vi "Initialization_T_B_ver1.1.vi"(1 "output cluster":T1={"Main Sweep"=0, "Steps Config:"={"total points:"=0, "Step Delay (s)"=0.0, "Ini Delay (s)"=0.0, "# of steps:"=0}, "Temperature Control (ITC 503):"={"GPIB ADR"=0, "Change Heater?"={"Heater?"=FALSE, "Heater"=0}, "Change Temp?"={"Change T?"=FALSE, "Set T (K)"=0.0}, "Cluster"={"Heat Auto?"=FALSE, "Manual Heat?"=FALSE, "Heater (%)"=0.0}, "Change PID?"={"Change PID?"=FALSE, "P"=0.0, "I"=0.0, "D"=0.0}, "Change Para?"=FALSE, "Sensor"=1}, "Temperature Control (LS 340):"={"GPIB ADR"=0, "From (K)"=0.0, "To (K)"=0.0, "Rate (K/min)"=0.0, "Delta T (0.08K)"=0.0, "Temp. Header"="", "T Display Control"={"Ch B"=FALSE, "Ch C"=FALSE, "Ch D"=FALSE}}, "Magnet Control (IPS 120-10)"={"Action"=0, "Standby (s)"=0.0, "Heater on (s)"=0.0, "Sweep Setup "=[], "GPIB ADR"=0, "Change Para?"=FALSE}, "Keithley 6221 :"=[], "Measuring Instruments : "=[], "Lock-In SR7265 :"=[], "Deascription of \nthis measurement"="", "Instruments Config:"=[], "LS372 Bridge : 2"=[{"GPIB"=0, "Excitation"=0, "Autorange?"=FALSE, "Range"=0, "Current"=0, "Voltage"=0, "DataHeader"="Rx;Ry"}], "Magnet Control (CS4) 2"={"Action"=1, "Standby (s)"=0.0, "Heater on (s)"=300.0, "Sweep Setup "=[], "GPIB ADR"=0, "Change Para?"=FALSE}} {"Magnet Control (CS4) 2"."GPIB ADR" items=["None"=0, "10"=10]; "Magnet Control (CS4) 2"."Sweep Setup"."Rate in Range (T/min)" min=0.001 max=0.5 step=0.001; "Magnet Control (CS4) 2"."Sweep Setup"."Hold(min)" min=0.0; "Magnet Control (CS4) 2"."Sweep Setup"."Set Point (T)" min=-9.0 max=9.0 step=0.001; "Magnet Control (CS4) 2"."Action" items=["Up", "Down", "Pause", "Zero"]; "LS372 Bridge : 2"."Voltage" items=["2.00 uV"=1, "6.32 uV"=2, "20.0 uV"=3, "63.2 uV"=4, "200 uV"=5, "632 uV"=6, "2.0 mV"=7, "6.32 mV"=8]; "LS372 Bridge : 2"."Current" items=["1.00 pA"=1, "3.16 pA"=2, "10.0 pA"=3, "31.6 pA"=4, "100 pA"=5, "316 pA"=6, "1.00 nA"=7, "3.16 nA"=8, "10 nA"=9, "31.6 nA"=10, "100 nA"=11, "316 nA"=12, "1.00 uA"=13, "3.16 uA"=14, "10.0 uA"=15, "31.6 uA"=16, "100 uA"=17, "316 uA"=18, "1.00 mA"=19, "3.16 mA"=20, "10.0 mA"=21, "31.6 mA"=22]; "LS372 Bridge : 2"."Range" items=["2.0 m"=1, "6.32 m"=2, "20.0 m"=3, "63.2 m"=4, "200 m"=5, "632 m"=6, "2.00"=7, "6.32"=8, "20.0"=9, "63.2"=10, "200"=11, "632"=12, "2.00 k"=13, "6.32 k"=14, "20.0 k"=15, "63.2 k"=16, "200 k"=17, "632 k"=18, "2.00 M"=19, "6.32 M"=20, "20.0 M"=21, "63.2 M"=22]; "LS372 Bridge : 2"."Excitation" items=["Voltage", "Current"]; "LS372 Bridge : 2"."GPIB" items=["None"=0, "9"=9]; "Main Sweep" items=["Time", "DC Current", "Delta Current", "Pulse Delta Current", "Sine Current", "Lock-in Vosc"]; "Temperature Control (ITC 503):"."Sensor" items=["T2", "T3"]; "Magnet Control (IPS 120-10)"."Action" items=["Hold", "To Set point", "To Zero", "Clamp"]; "Keithley 6221 :"."Sweep Mode" items=["Linear", "Log", "Exp", "Inverse", "Manual"]}, 5 "Measure with H/T sweep?":bool, 6 "error in (no error)":errorcluster, 7 "First run?":bool, 8 "Last run?":bool, 9 "B Field Display Tex Array":refnum<vi>[](array[refnum]), 10 "Temp. Display Ref Array":refnum<vi>[](array[refnum])) -> (0 "error out":errorcluster, 2 "output cluster 2":T1={"Main Sweep"=0, "Steps Config:"={"total points:"=0, "Step Delay (s)"=0.0, "Ini Delay (s)"=0.0, "# of steps:"=0}, "Temperature Control (ITC 503):"={"GPIB ADR"=0, "Change Heater?"={"Heater?"=FALSE, "Heater"=0}, "Change Temp?"={"Change T?"=FALSE, "Set T (K)"=0.0}, "Cluster"={"Heat Auto?"=FALSE, "Manual Heat?"=FALSE, "Heater (%)"=0.0}, "Change PID?"={"Change PID?"=FALSE, "P"=0.0, "I"=0.0, "D"=0.0}, "Change Para?"=FALSE, "Sensor"=1}, "Temperature Control (LS 340):"={"GPIB ADR"=0, "From (K)"=0.0, "To (K)"=0.0, "Rate (K/min)"=0.0, "Delta T (0.08K)"=0.0, "Temp. Header"="", "T Display Control"={"Ch B"=FALSE, "Ch C"=FALSE, "Ch D"=FALSE}}, "Magnet Control (IPS 120-10)"={"Action"=0, "Standby (s)"=0.0, "Heater on (s)"=0.0, "Sweep Setup "=[], "GPIB ADR"=0, "Change Para?"=FALSE}, "Keithley 6221 :"=[], "Measuring Instruments : "=[], "Lock-In SR7265 :"=[], "Deascription of \nthis measurement"="", "Instruments Config:"=[], "LS372 Bridge : 2"=[{"GPIB"=0, "Excitation"=0, "Autorange?"=FALSE, "Range"=0, "Current"=0, "Voltage"=0, "DataHeader"="Rx;Ry"}], "Magnet Control (CS4) 2"={"Action"=1, "Standby (s)"=0.0, "Heater on (s)"=300.0, "Sweep Setup "=[], "GPIB ADR"=0, "Change Para?"=FALSE}} {"Magnet Control (CS4) 2"."GPIB ADR" items=["None"=0, "25"=25]; "Magnet Control (CS4) 2"."Sweep Setup"."Rate in Range (T/min)" min=0.001 max=0.5 step=0.001; "Magnet Control (CS4) 2"."Sweep Setup"."Hold(min)" min=0.0; "Magnet Control (CS4) 2"."Sweep Setup"."Set Point (T)" min=-9.0 max=9.0 step=0.001; "Magnet Control (CS4) 2"."Action" items=["Up", "Down", "Pause", "Zero"]; "LS372 Bridge : 2"."Voltage" items=["2.00 uV"=1, "6.32 uV"=2, "20.0 uV"=3, "63.2 uV"=4, "200 uV"=5, "632 uV"=6, "2.0 mV"=7, "6.32 mV"=8]; "LS372 Bridge : 2"."Current" items=["1.00 pA"=1, "3.16 pA"=2, "10.0 pA"=3, "31.6 pA"=4, "100 pA"=5, "316 pA"=6, "1.00 nA"=7, "3.16 nA"=8, "10 nA"=9, "31.6 nA"=10, "100 nA"=11, "316 nA"=12, "1.00 uA"=13, "3.16 uA"=14, "10.0 uA"=15, "31.6 uA"=16, "100 uA"=17, "316 uA"=18, "1.00 mA"=19, "3.16 mA"=20, "10.0 mA"=21, "31.6 mA"=22]; "LS372 Bridge : 2"."Range" items=["2.0 m"=1, "6.32 m"=2, "20.0 m"=3, "63.2 m"=4, "200 m"=5, "632 m"=6, "2.00"=7, "6.32"=8, "20.0"=9, "63.2"=10, "200"=11, "632"=12, "2.00 k"=13, "6.32 k"=14, "20.0 k"=15, "63.2 k"=16, "200 k"=17, "632 k"=18, "2.00 M"=19, "6.32 M"=20, "20.0 M"=21, "63.2 M"=22]; "LS372 Bridge : 2"."Excitation" items=["Voltage", "Current"]; "LS372 Bridge : 2"."GPIB" items=["None"=0, "9"=9]; "Main Sweep" items=["Time", "DC Current", "Delta Current", "Pulse Delta Current", "Sine Current", "Lock-in Vosc"]; "Temperature Control (ITC 503):"."Sensor" items=["T2", "T3"]; "Magnet Control (IPS 120-10)"."Action" items=["Hold", "To Set point", "To Zero", "Clamp"]; "Keithley 6221 :"."Sweep Mode" items=["Linear", "Log", "Exp", "Inverse", "Manual"]}, 3 "Title Array":string[](array[string]), 4 "Comments String":string)   [LabVIEW 2012]
doc: "Initialize the temperature (LS336)"
panel:
  out "BField Display Cluster":cluster{"B":dbl} {"B" min=0.0 format="%_5f"}
  out "B Set Pt (T)":dbl format="%_5g"
  out "B Rate (T/min)":dbl format="%_5g"
  out "Temp Graph 2":dbl[][](graph)=[[348.0650696299951, 348.0650696299951, 348.0650696299951, 348.0650696299951, 348.0650696299951, 348.0650696299951, 348.0650696299951, 348.0650696299951, 348.0650696299951, 348.0650696299951, 348.0650696299951, 348.0650696299951, 348.0650696299951, 348.0650696299951, 348.0650696299951], [349.0, 349.0, 349.0, 349.0, 349.0, 349.0, 349.0, 349.0, 349.0, 349.0, 349.0, 349.0, 349.0, 349.0, 349.0], [347.994, 347.998, 348.007, 348.013, 348.031, 348.047, 348.071, 348.073, 348.076, 348.088, 348.106, 348.11, 348.113, 348.121, 348.128], [349.08, 349.08, 349.08, 349.08, 349.08, 349.08, 349.08, 349.08, 349.08, 349.08, 349.08, 349.08, 349.08, 349.08, 349.08], [348.92, 348.92, 348.92, 348.92, 348.92, 348.92, 348.92, 348.92, 348.92, 348.92, 348.92, 348.92, 348.92, 348.92, 348.92]]
  out "StartTime":u32
  in  "Skip":bool
  out "Time 2":string
  in  "Timeout (min)":u32=30
  out "Reach to set pt?":bool
  out "T Rate (K/min)":dbl format="%_5g"
  out "T Set Pt (K)":dbl format="%_5g"
  out "Temp Display Cluster":cluster{"RMS T:":dbl, "T STD":dbl, "T":dbl} {"T STD" min=0.0 format="%8.4f"; "T" min=0.0 format="%_5f"; "RMS T:" format="%_5g"}
  out "Temp Graph":dbl[][](graph)=[[348.0650696299951, 348.0650696299951, 348.0650696299951, 348.0650696299951, 348.0650696299951, 348.0650696299951, 348.0650696299951, 348.0650696299951, 348.0650696299951, 348.0650696299951, 348.0650696299951, 348.0650696299951, 348.0650696299951, 348.0650696299951, 348.0650696299951], [349.0, 349.0, 349.0, 349.0, 349.0, 349.0, 349.0, 349.0, 349.0, 349.0, 349.0, 349.0, 349.0, 349.0, 349.0], [347.994, 347.998, 348.007, 348.013, 348.031, 348.047, 348.071, 348.073, 348.076, 348.088, 348.106, 348.11, 348.113, 348.121, 348.128], [349.08, 349.08, 349.08, 349.08, 349.08, 349.08, 349.08, 349.08, 349.08, 349.08, 349.08, 349.08, 349.08, 349.08, 349.08], [348.92, 348.92, 348.92, 348.92, 348.92, 348.92, 348.92, 348.92, 348.92, 348.92, 348.92, 348.92, 348.92, 348.92, 348.92]]
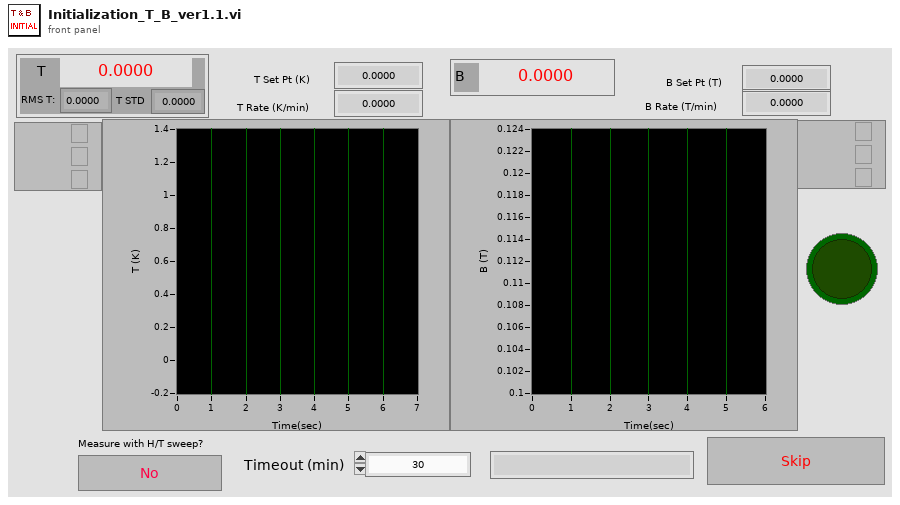
[diagram p1: front panel]
types:
  T1 = cluster{"Main Sweep":u8, "Steps Config:":cluster{"total points:":u32, "Step Delay (s)":dbl, "Ini Delay (s)":dbl, "# of steps:":u32}, "Temperature Control (ITC 503):":cluster{"GPIB ADR":u16, "Change Heater?":cluster{"Heater?":bool, "Heater":u8}, "Change Temp?":cluster{"Change T?":bool, "Set T (K)":dbl}, "Cluster":cluster{"Heat Auto?":bool, "Manual Heat?":bool, "Heater (%)":dbl}, "Change PID?":cluster{"Change PID?":bool, "P":dbl, "I":dbl, "D":dbl}, "Change Para?":bool, "Sensor":u16}, "Temperature Control (LS 340):":cluster{"GPIB ADR":u16, "From (K)":dbl, "To (K)":dbl, "Rate (K/min)":dbl, "Delta T (0.08K)":dbl, "Temp. Header":string, "T Display Control":cluster{"Ch B":bool, "Ch C":bool, "Ch D":bool}}, "Magnet Control (IPS 120-10)":cluster{"Action":u16, "Standby (s)":dbl, "Heater on (s)":dbl, "Sweep Setup ":cluster{"Set Point (T)":dbl, "Set Rate(T/min)":dbl, "Hold(min)":dbl}[], "GPIB ADR":u16, "Change Para?":bool}, "Keithley 6221 :":cluster{"Delta mode":bool, "Const I":bool, "Pulse Delta mode":bool, "Sine Wave Mode":bool, "From I_HI (A)":dbl, "From I (A)":dbl, "I_LO (A)":dbl, "From I_H (A)":dbl, "I_L (A)":dbl, "Freq (Hz)":dbl, "From I_Sin (A)":dbl, "DC Offset (A)":dbl, "Delay Time (s)":dbl, "Pulse Width (s)":dbl, "Delay (s)":dbl, "To I (A)":dbl, "ASymmetric?":bool, "To I_HI (A)":dbl, "To I_H (A)":dbl, "To I_Sin (A)":dbl, "GPIB ADR":u16, "Sweep Mode":u8, "Delta Unit":string, "2182A range (V)":dbl, "6221 Compliance (V)":dbl}[], "Measuring Instruments : ":cluster{"GPIB Bus":dbl, "GPIB Addr":dbl, "Instrument":enum16{"None", "HP34401DMM", "Lockin 7265", "HP3456/7A", "HP3478A", "HP3325FG", "Keithley2182A"}, "Instru Header":string}[], "Lock-In SR7265 :":cluster{"GPIB ADR":u16, "From":dbl, "To":dbl, "Header(;)":string, "Sweep Mode":u8}[], "Deascription of \nthis measurement":string, "Instruments Config:":string[][], "LS372 Bridge : 2":cluster{"GPIB":u16, "Excitation":u16, "Autorange?":bool, "Range":u16, "Current":u16, "Voltage":u16, "DataHeader":string}[], "Magnet Control (CS4) 2":cluster{"Action":u16, "Standby (s)":dbl, "Heater on (s)":dbl, "Sweep Setup ":cluster{"Set Point (T)":dbl, "Hold(min)":dbl, "Rate in Range (T/min)":dbl[]}[], "GPIB ADR":u16, "Change Para?":bool}}
  T2 = cluster{"GPIB ADR":u16, "Change Heater?":cluster{"Heater?":bool, "Heater":u8}, "Change Temp?":cluster{"Change T?":bool, "Set T (K)":dbl}, "Cluster":cluster{"Heat Auto?":bool, "Manual Heat?":bool, "Heater (%)":dbl}, "Change PID?":cluster{"Change PID?":bool, "P":dbl, "I":dbl, "D":dbl}, "Change Para?":bool, "Sensor":u16}
  T3 = cluster{"Action":u16, "Standby (s)":dbl, "Heater on (s)":dbl, "Sweep Setup ":cluster{"Set Point (T)":dbl, "Set Rate(T/min)":dbl, "Hold(min)":dbl}[], "GPIB ADR":u16, "Change Para?":bool}
  T4 = cluster{"GPIB ADR":u16, "From (K)":dbl, "To (K)":dbl, "Rate (K/min)":dbl, "Delta T (0.08K)":dbl, "Temp. Header":string, "T Display Control":cluster{"Ch B":bool, "Ch C":bool, "Ch D":bool}}
  T5 = cluster{"Action":u16, "Standby (s)":dbl, "Heater on (s)":dbl, "Sweep Setup ":cluster{"Set Point (T)":dbl, "Hold(min)":dbl, "Rate in Range (T/min)":dbl[]}[], "GPIB ADR":u16, "Change Para?":bool}
  T6 = cluster{"RMS":dbl, "STD":dbl, "Current value":dbl}
  T7 = cluster{"Com Port":i32, "ISOBUS Address":i32, "GPIB Address":i16, "Communication":enum16{"RS232", "ISOBUS", "GPIB", "Gateway"}}
  T8 = cluster{"GPIB ADR":u16, "Change Heater?":cluster{"Change Heater?":bool, "Heater":u8}, "Change Temp?":cluster{"Change Temp?":bool, "Set Temp (K)":dbl}, "Cluster":cluster{"Heat Auto?":bool, "Manual Heat?":bool, "Heater Manual (%)":dbl}, "Change PID?":cluster{"Change PID?":bool, "Proportional":dbl, "Integral":dbl, "Derivative":dbl}, "Change Para?":bool, "ITC503 Control Sensor":u16}
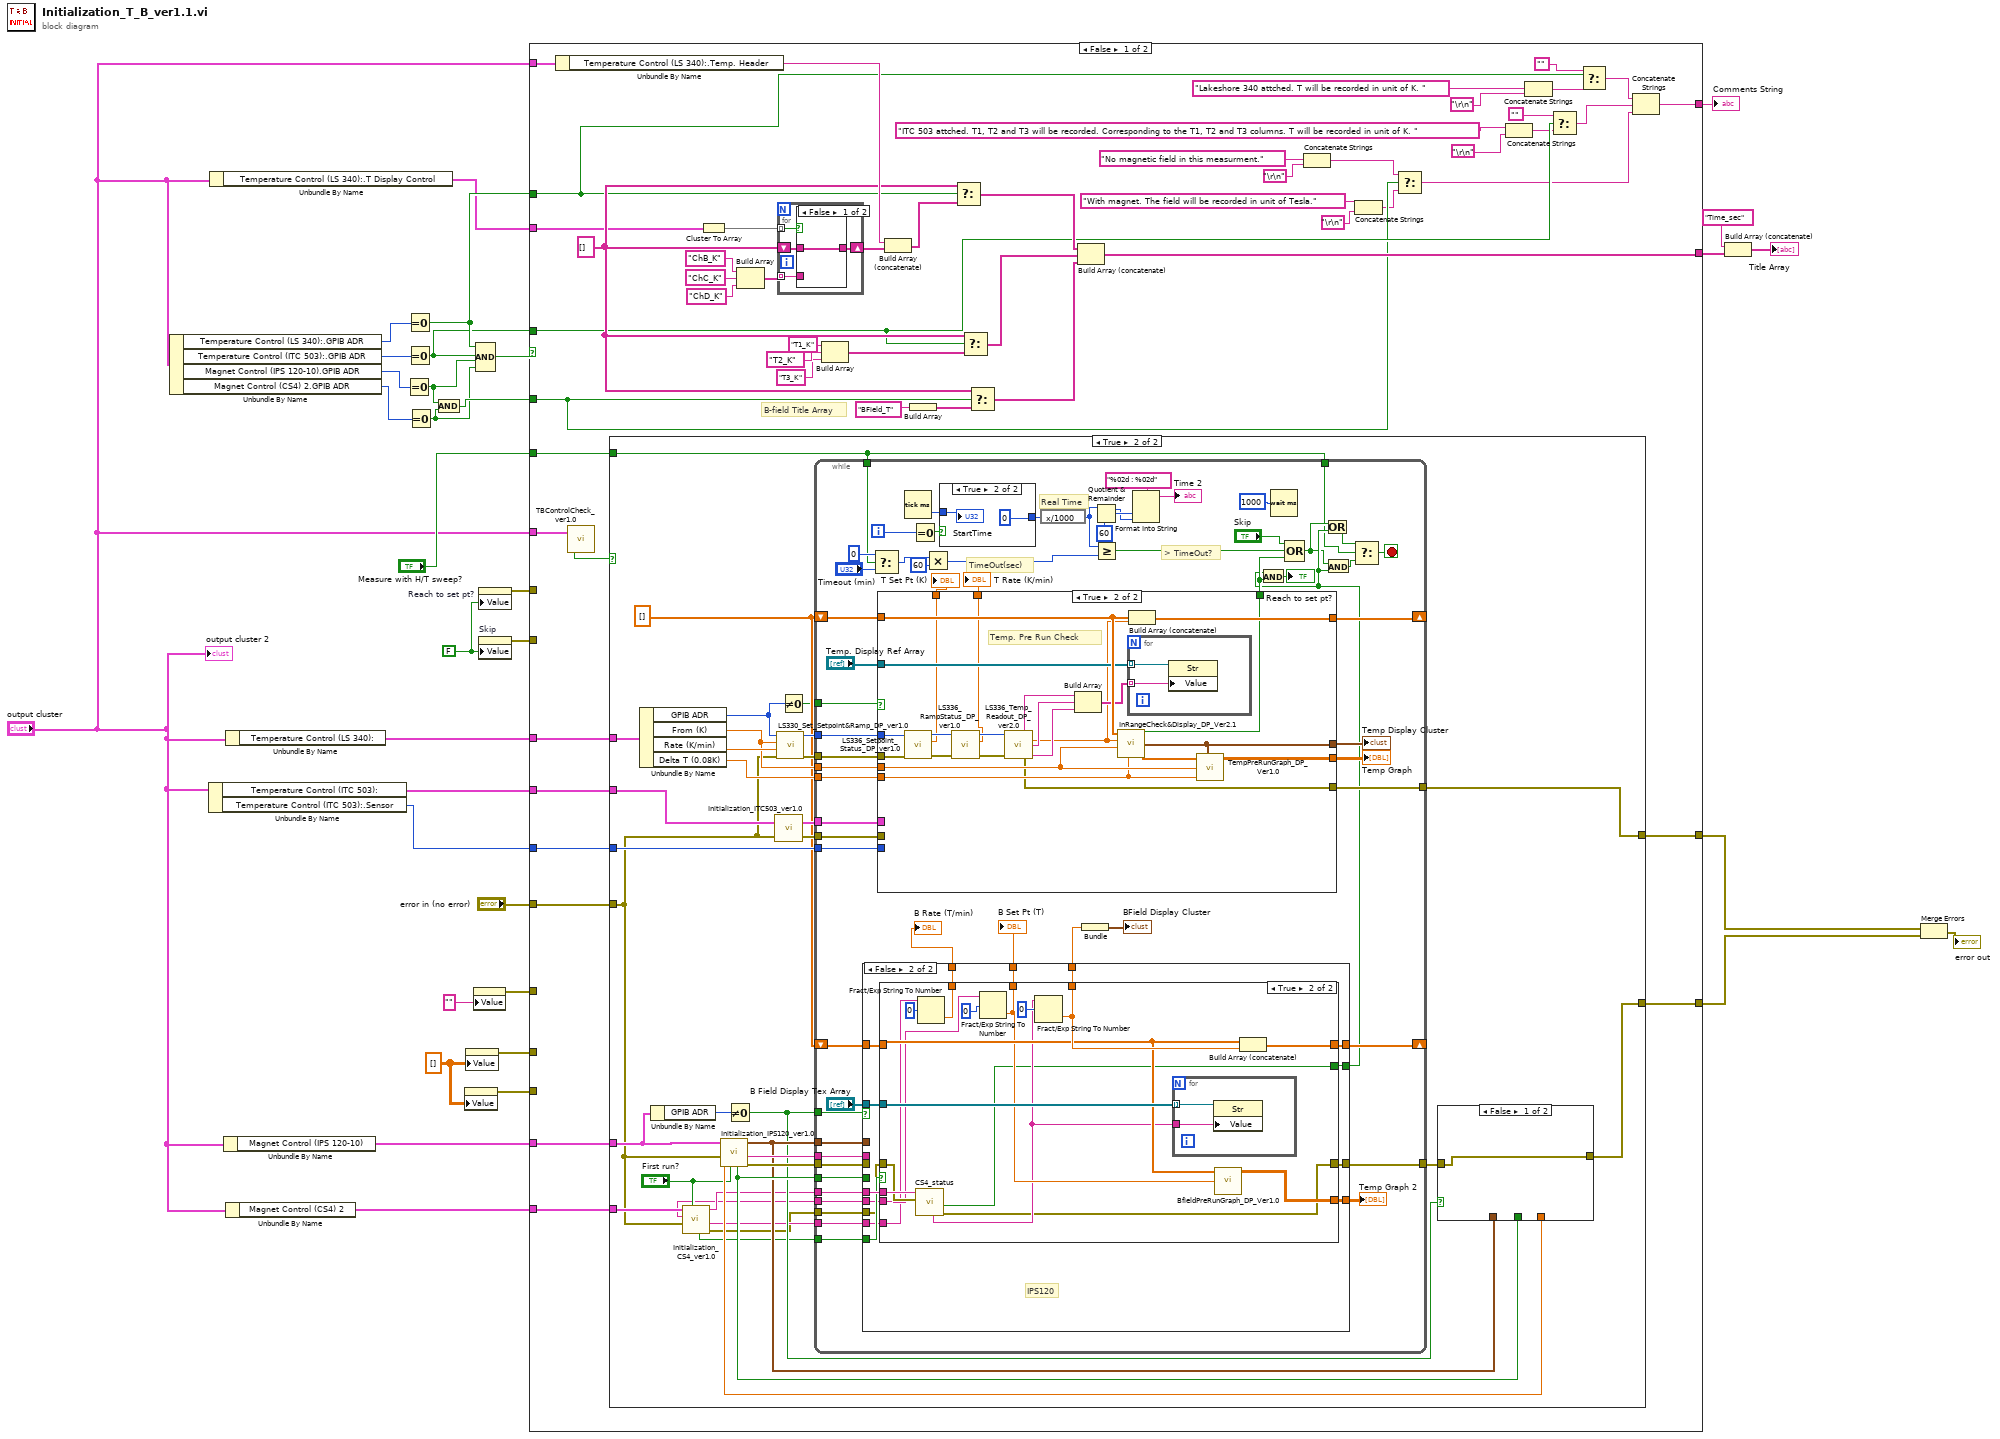
[diagram p0: block diagram]
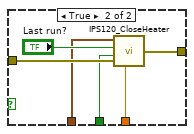
[diagram p3: hidden frame]
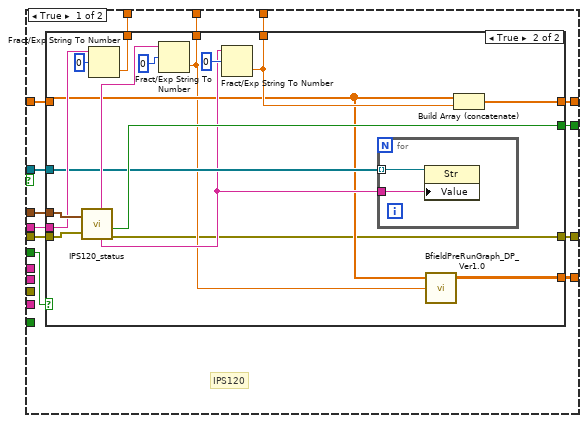
[diagram p4: hidden frame]
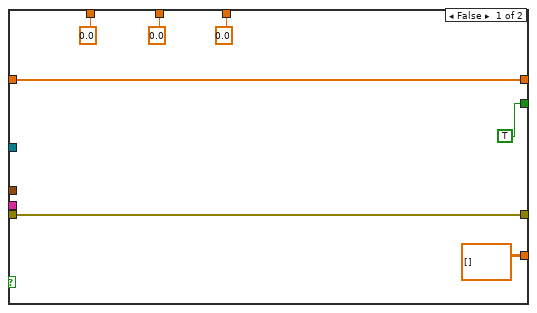
[diagram p5: hidden frame]
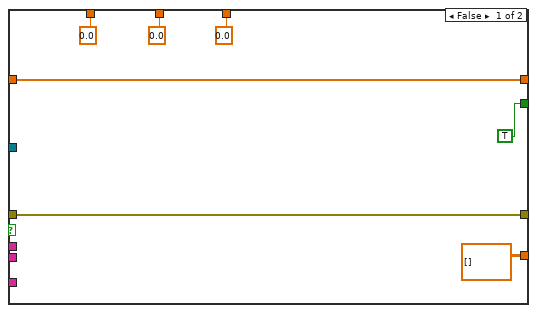
[diagram p6: hidden frame]
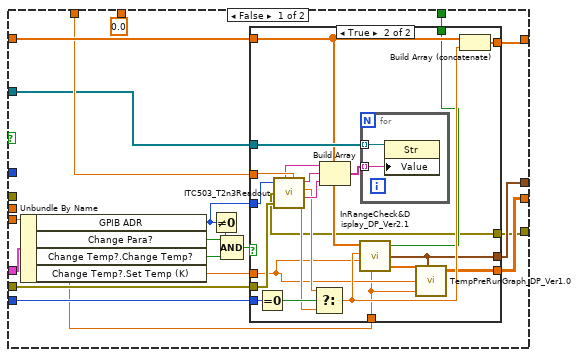
[diagram p7: hidden frame]
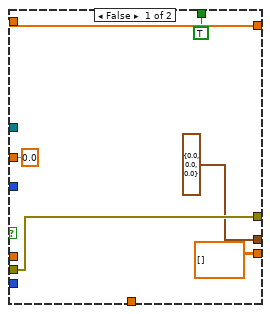
[diagram p8: hidden frame]
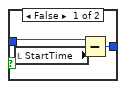
[diagram p9: hidden frame]
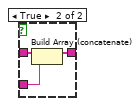
[diagram p10: hidden frame]
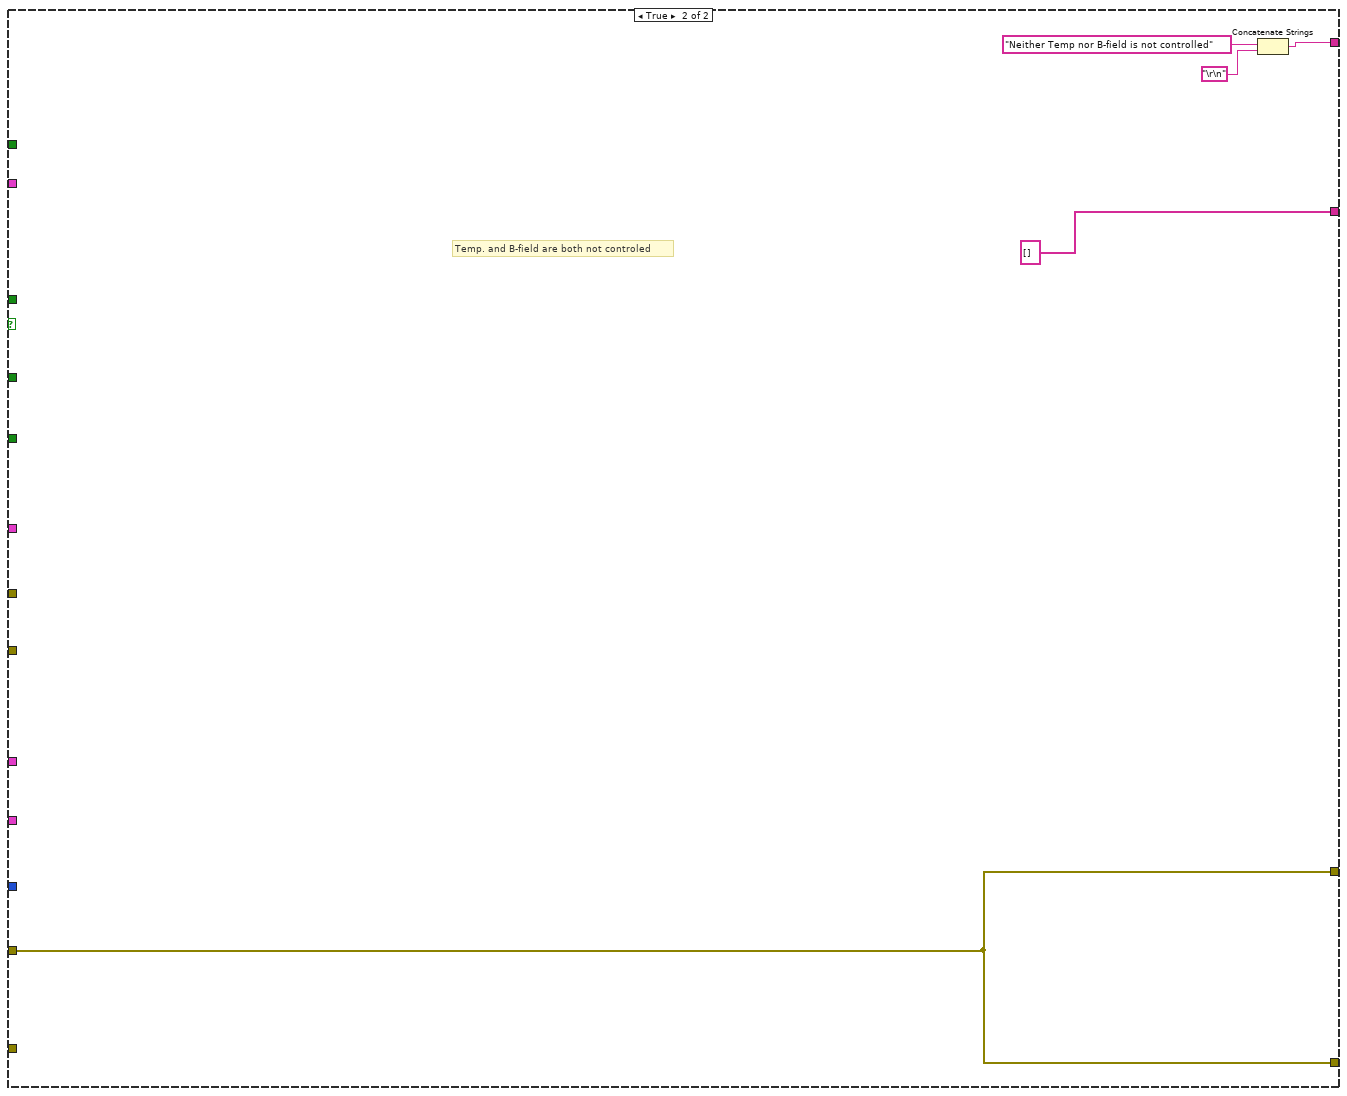
[diagram p11: hidden frame]
diagram:
  w10 = FALSE ("Skip")
  w17 = dbl[][] []
  n1 = Unbundle By Name("output cluster") -> ("Temperature Control (LS 340):.GPIB ADR"=w34:u16, "Temperature Control (ITC 503):.GPIB ADR"=w33:u16, "Magnet Control (IPS 120-10).GPIB ADR"=w32:u16, "Magnet Control (CS4) 2.GPIB ADR"=w4:u16)
  n2 = Unbundle By Name("output cluster") -> ("Temperature Control (ITC 503):"=w20:T2, "Temperature Control (ITC 503):.Sensor"=w9:u16)
  n3 = Unbundle By Name("output cluster") -> ("Temperature Control (LS 340):.T Display Control"=w18:cluster{"Ch B":bool, "Ch C":bool, "Ch D":bool})
  n4 = Unbundle By Name("output cluster") -> ("Magnet Control (IPS 120-10)"=w5:T3)
  n5 = Unbundle By Name("output cluster") -> ("Temperature Control (LS 340):"=w21:T4)
  n6 = Unbundle By Name("output cluster") -> ("Magnet Control (CS4) 2"=w6:T5)
  n7 = Equal To 0?(x=w32) -> (x = 0?=w3:bool)
  n8 = Equal To 0?(x=w34) -> (x = 0?=w23:bool)
  n9 = Equal To 0?(x=w33) -> (x = 0?=w22:bool)
  n10 = Equal To 0?(x=w4) -> (x = 0?=w1:bool)
  n11 = And(x=w3, y=w1) -> (x .and. y?=w2:bool)
  n12 = property on="Temp Graph 2" class="WFGraph (strict)"("Value"=w17) -> (error out=w15:errorcluster)  [unwired: 2 in, 1 out]
  n13 = property on="Temp Graph" class="WFGraph (strict)"("Value"=w17) -> (error out=w16:errorcluster)  [unwired: 2 in, 1 out]
  n14 = property on="Time 2" class="Str"("Value"="" ("Time 2")) -> (error out=w13:errorcluster)  [unwired: 2 in, 1 out]
  n15 = Compound Arithmetic op=AND(w23, w22, w3, w1) -> (w31:bool)
  n16 = property on="Reach to set pt?" class="Bool (strict)"("Value"=w10) -> (error out=w11:errorcluster)  [unwired: 2 in, 1 out]
  n17 = property on="Skip" class="Bool (strict)"("Value"=w10) -> (error out=w12:errorcluster)  [unwired: 2 in, 1 out]
  n18 = case shown="False" w31 {
    tunnel: [w78 string[] []] -> w29
    tunnel: "error in (no error)" -> [w68 w360]
    tunnel: [w67 w360] -> w25
    tunnel: [w66 w360] -> w24
    tunnel: w23 -> [w63 _]
    tunnel: w22 -> [w58 _]
    tunnel: w2 -> [w50 _]
    tunnel: w21 -> [w65 _]
    tunnel: w20 -> [w37 _]
    tunnel: w5 -> [w36 _]
    tunnel: [w44 w357] -> w19
    tunnel: w18 -> [w43 _]
    tunnel: w9 -> [w42 _]
    tunnel: w16 -> [_ _]
    tunnel: w15 -> [_ _]
    tunnel: w13 -> [_ _]
    tunnel: w12 -> [_ _]
    tunnel: w11 -> [_ _]
    tunnel: "Measure with H/T sweep?" -> [w41 _]
    tunnel: "output cluster" -> [w39 _]
    tunnel: "output cluster" -> [w38 _]
    tunnel: w6 -> [w35 _]
    frame False {
      w73 = string[] []
      # "B-field Title Array"
      n19 = Unbundle By Name(w39) -> ("Temperature Control (LS 340):.Temp. Header"=w81:string)
      n20 = call "TBControlCheck_ver1.0.vi"("output cluster"=w38) -> ("T&B Setting Change?"=w69:bool)  [unwired: 3 out]
      n21 = case shown="True" w69 {
        tunnel: w68 -> [w88 w95]
        tunnel: [w88 w113] -> w67
        tunnel: [w88 w107] -> w66
        tunnel: w65 -> [_ w120]
        tunnel: w37 -> [_ w121]
        tunnel: w36 -> [_ w101]
        tunnel: w42 -> [_ w111]
        tunnel: w41 -> [_ w102]
        tunnel: w35 -> [_ w96]
        frame False {
          # "T and B settings are not changed"
        }
        frame True {
          w108 = dbl[] []
          n22 = Unbundle By Name(w120) -> ("GPIB ADR"=w100:u16, "From (K)"=w116:dbl, "Rate (K/min)"=w119:dbl, "Delta T (0.08K)"=w115:dbl)
          n23 = Unbundle By Name(w101) -> ("GPIB ADR"=w98:u16)
          n24 = call "Initialization_CS4_ver1.0.vi"("Magnet Control (CS4)"=w96, "error in"=w95, "First run?"="First run?") -> ("Set point"=w91:string, "B field Change?"=w92:bool, "GPIB adr"=w93:string, "Rate"=w90:string, "error out"=w89:errorcluster)  [unwired: 1 in, 2 out]
          n25 = call "Initialization_IPS120_ver1.0.vi"("Magnet Control (IPS 120-10)"=w101, "error in"=w95, "First run?"="First run?") -> ("Hold(min)"=w103:dbl, "B field Change?"=w105:bool, "output cluster"=w104:T7, "Rate"=w109:string, "error out"=w110:errorcluster)  [unwired: 3 out]
          n26 = Not Equal To 0?(x=w98) -> (x != 0?=w94:bool)
          n27 = call "Initialization_ITC503_ver1.0.vi"("error in"=w95, "Temperature Control (ITC 503):"=w121) -> ("error out"=w114:errorcluster, "Temperature Control (ITC 503): 2"=w112:T8)
          n28 = call "LS330_Set_Setpoint&Ramp_DP_ver1.0.vi"("error in"=w95, "Ramping rate (0-100 K/min; 1.0)"=w119, "Setpoint (2-400 K)"=w116, "GPIB ADR (19)"=w100) -> ("error out"=w117:errorcluster, "dump GPIB ADR"=w118:i16)  [unwired: 6 in]
          n29 = Not Equal To 0?(x=w100) -> (x != 0?=w99:bool)
          n30 = while {
            tunnel: w118 -> [w173]
            tunnel: w117 -> [w172]
            shift-right: [w174] -> _
            shift-left: w108 -> [w175]
            tunnel: w116 -> [w171]
            tunnel: w115 -> [w170]
            tunnel: w114 -> [w163]
            tunnel: [w162] -> w113
            tunnel: w112 -> [w161]
            tunnel: w111 -> [w160]
            tunnel: w105 -> [w159]
            tunnel: w104 -> [w158]
            tunnel: w110 -> [w157]
            tunnel: w109 -> [w156]
            shift-right: [w150] -> _
            shift-left: w108 -> [w151]
            tunnel: [w147] -> w106
            tunnel: w102 -> [w140]
            tunnel: w102 -> [w136]
            tunnel: w99 -> [w135]
            tunnel: w94 -> [w134]
            tunnel: w93 -> [w133]
            tunnel: w92 -> [w132]
            tunnel: w91 -> [w131]
            tunnel: w90 -> [w130]
            tunnel: w89 -> [w129]
            i -> [w178]
            stop <- w141 stop-if-true
            # "Real Time"
            # "> TimeOut?"
            # "TimeOut(sec)"
            n31 = case shown="False" w134 {
              tunnel: w159 -> [w203 _]
              tunnel: w158 -> [w202 _]
              tunnel: w157 -> [w201 _]
              tunnel: w156 -> [w200 _]
              tunnel: [w199 w243] -> w155
              tunnel: [w198 w242] -> w154
              tunnel: [w197 w241] -> w153
              tunnel: w151 -> [w196 w240]
              tunnel: [w195 w239] -> w150
              tunnel: "B Field Display Tex Array" -> [w194 w238]
              tunnel: [w193 w237] -> w148
              tunnel: [w192 w236] -> w147
              tunnel: [w191 w235] -> w145
              tunnel: w133 -> [_ w234]
              tunnel: w132 -> [_ w233]
              tunnel: w131 -> [_ w232]
              tunnel: w130 -> [_ w231]
              tunnel: w129 -> [_ w230]
              frame True {
                # "IPS120"
                n32 = case shown="True" w203 {
                  tunnel: [TRUE ("B field change stop") w225] -> w191
                  tunnel: w202 -> [_ w227]
                  tunnel: w201 -> [w204 w226]
                  tunnel: w200 -> [_ w224]
                  tunnel: [0.0 w222] -> w199
                  tunnel: [0.0 w213] -> w198
                  tunnel: [0.0 w217] -> w197
                  tunnel: w196 -> [w209 w214]
                  tunnel: [w209 w218] -> w195
                  tunnel: w194 -> [_ w216]
                  tunnel: [dbl[][] [] ("BField Graph") w212] -> w193
                  tunnel: [w204 w211] -> w192
                  frame False {
                  }
                  frame True {
                    n33 = call "IPS120_status.vi"("Address"=w227, "error in"=w226) -> ("Set point"=w220:string, "Real Field"=w215:string, "Arrive"=w225:bool, "error out"=w211:errorcluster)  [unwired: 2 out]
                    n34 = Fract/Exp String To Number(string=w224, offset=0) -> (number=w222:dbl)  [unwired: 2 in, 1 out]
                    n35 = Fract/Exp String To Number(string=w220, offset=0) -> (number=w213:dbl)  [unwired: 2 in, 1 out]
                    n36 = Fract/Exp String To Number(string=w215, offset=0) -> (number=w217:dbl)  [unwired: 2 in, 1 out]
                    n37 = for {
                      tunnel: w215 -> [w228]
                      tunnel: w216 -> [w229] mode=indexing
                      n38 = property class="Str"(reference=w229, "Value"=w228) -> ()  [unwired: 1 in, 2 out]
                    }
                    n39 = call "BfieldPreRunGraph_DP_Ver1.0.vi"("B Array"=w214, "Set Pt"=w213) -> ("BField Graph"=w212:dbl[][])  [unwired: 5 in]
                    n40 = Build Array (concatenate)(w214, w217) -> (w218:dbl[])
                  }
                }
              }
              frame False {
                # "IPS120"
                n41 = case shown="True" w233 {
                  tunnel: [TRUE ("B field change stop") w251] -> w235
                  tunnel: [0.0 w266] -> w243
                  tunnel: [0.0 w259] -> w242
                  tunnel: [0.0 w262] -> w241
                  tunnel: w240 -> [w249 w260]
                  tunnel: [w249 w263] -> w239
                  tunnel: w238 -> [_ w261]
                  tunnel: [dbl[][] [] ("BField Graph") w258] -> w237
                  tunnel: [w244 w252] -> w236
                  tunnel: w234 -> [_ w257]
                  tunnel: w230 -> [w244 w256]
                  tunnel: w232 -> [_ w254]
                  tunnel: w231 -> [_ w253]
                  frame False {
                  }
                  frame True {
                    n42 = call "CS4_status.vi"("address string"=w257, "error in"=w256) -> ("Real Field"=w255:string, "Arrive"=w251:bool, "error out"=w252:errorcluster)  [unwired: 6 out]
                    n43 = Fract/Exp String To Number(string=w253, offset=0) -> (number=w266:dbl)  [unwired: 2 in, 1 out]
                    n44 = Fract/Exp String To Number(string=w254, offset=0) -> (number=w259:dbl)  [unwired: 2 in, 1 out]
                    n45 = Fract/Exp String To Number(string=w255, offset=0) -> (number=w262:dbl)  [unwired: 2 in, 1 out]
                    n46 = for {
                      tunnel: w255 -> [w268]
                      tunnel: w261 -> [w269] mode=indexing
                      n47 = property class="Str"(reference=w269, "Value"=w268) -> ()  [unwired: 1 in, 2 out]
                    }
                    n48 = call "BfieldPreRunGraph_DP_Ver1.0.vi"("B Array"=w260, "Set Pt"=w259) -> ("BField Graph"=w258:dbl[][])  [unwired: 5 in]
                    n49 = Build Array (concatenate)(w260, w262) -> (w263:dbl[])
                  }
                }
              }
            }
            "B Set Pt (T)" <- w154
            "B Rate (T/min)" <- w155
            "Temp Graph 2" <- w148
            n50 = Select(t=u32 0, s=w136, f="Timeout (min)") -> (s? t:f=w138:u32)
            n51 = case shown="True" w135 {
              tunnel: w175 -> [w287 w331]
              tunnel: [w286 w341] -> w174
              tunnel: w173 -> [_ w340]
              tunnel: w172 -> [_ w339]
              tunnel: w171 -> [_ w329]
              tunnel: w170 -> [w274 w328]
              tunnel: [w271 w327] -> w146
              tunnel: "Temp. Display Ref Array" -> [w276 w325]
              tunnel: [w270 w324] -> w162
              tunnel: [w278 w322] -> w167
              tunnel: [0.0 ("Ramp Rate") w321] -> w166
              tunnel: [w272 w320] -> w165
              tunnel: [w273 w319] -> w164
              tunnel: w163 -> [w288 _]
              tunnel: w161 -> [w285 _]
              tunnel: w160 -> [w275 _]
              frame False {
                n52 = Unbundle By Name(w285) -> ("GPIB ADR"=w280:u16, "Change Para?"=w282:bool, "Change Temp?.Change Temp?"=w281:bool, "Change Temp?.Set Temp (K)"=w279:dbl)
                n53 = Not Equal To 0?(x=w280) -> (x != 0?=w283:bool)
                n54 = Compound Arithmetic op=AND(w283, w282, w281) -> (w284:bool)
                n55 = case shown="True" w284 {
                  tunnel: w288 -> [w292 w316]
                  tunnel: w287 -> [w294 w303]
                  tunnel: [w294 w315] -> w286
                  tunnel: w280 -> [_ w314]
                  tunnel: w279 -> [_ w298]
                  tunnel: [0.0 ("Set T") w313] -> w278
                  tunnel: w276 -> [_ w309]
                  tunnel: w275 -> [_ w307]
                  tunnel: w274 -> [_ w297]
                  tunnel: [T6 {"RMS"=0.0, "STD"=0.0, "Current value"=0.0} ("Display Cluster") w300] -> w273
                  tunnel: [dbl[][] [] ("Temp Graph") w299] -> w272
                  tunnel: [TRUE ("Reach to set pt?") w296] -> w271
                  tunnel: [w292 w295] -> w270
                  frame False {
                  }
                  frame True {
                    n56 = Equal To 0?(x=w307) -> (x = 0?=w306:bool)
                    n57 = call "ITC503_T2n3Readout.vi"("GPIB Address"=w314, "error in"=w316) -> ("error out"=w295:errorcluster, "Sensor T1"=w312:string, "Set T"=w313:dbl, "Sensor T2"=w311:string, "T2"=w305:dbl, "Sensor T3"=w310:string, "T3"=w304:dbl)  [unwired: 2 out]
                    n58 = Select(t=w305, s=w306, f=w304) -> (s? t:f=w302:dbl)
                    n59 = Build Array(w312, w311, w310) -> (w308:string[])
                    n60 = call "InRangeCheck&Display_DP_Ver2.1.vi"("Delta range>0"=w297, "Set Point"=w298, "Current value"=w302, "Data Array In"=w303) -> ("Data Array Out"=w301:dbl[], "Display Cluster"=w300:T6, "Reach to set pt?"=w296:bool)  [unwired: 4 in]
                    n61 = for {
                      tunnel: w308 -> [w317] mode=indexing
                      tunnel: w309 -> [w318] mode=indexing
                      n62 = property class="Str"(reference=w318, "Value"=w317) -> ()  [unwired: 1 in, 2 out]
                    }
                    n63 = call "TempPreRunGraph_DP_Ver1.0.vi"("T Array"=w301, "Temp Display Cluster (Need RMS)"=w300, "Set Pt"=w298, "Delta T"=w297) -> ("Temp Graph"=w299:dbl[][])  [unwired: 3 in]
                    n64 = Build Array (concatenate)(w303, w302) -> (w315:dbl[])
                  }
                }
              }
              frame True {
                # "Temp. Pre Run Check"
                n65 = call "LS336_Setpoint_Status_DP_ver1.0.vi"("error in"=w339, "GPIB ADR (18)"=w340) -> ("error out"=w337:errorcluster, "Setpoint"=w322:dbl, "dump GPIB ADR"=w338:i16)  [unwired: 2 in, 1 out]
                n66 = call "LS336_RampStatus_DP_ver1.0.vi"("GPIB ADR (18)"=w338, "error in"=w337) -> ("dump GPIB ADR"=w336:i16, "Ramp Rate"=w321:dbl, "error out"=w335:errorcluster)  [unwired: 2 in, 3 out]
                n67 = call "LS336_Temp_Readout_DP_ver2.0.vi"("GPIB ADR (18)"=w336, "error in"=w335) -> (2:"Sensor A (K)"=w323:dbl, 3:"Sensor A (K)"=w334:string, "Sensor B (K)"=w333:string, "error out"=w324:errorcluster, "Sensor C (K)"=w332:string)  [unwired: 4 in, 5 out]
                n68 = Build Array(w334, w333, w332) -> (w326:string[])
                n69 = call "InRangeCheck&Display_DP_Ver2.1.vi"("Delta range>0"=w328, "Set Point"=w329, "Current value"=w323, "Data Array In"=w331) -> ("Data Array Out"=w330:dbl[], "Display Cluster"=w319:T6, "Reach to set pt?"=w327:bool)  [unwired: 4 in]
                n70 = for {
                  tunnel: w326 -> [w342] mode=indexing
                  tunnel: w325 -> [w343] mode=indexing
                  n71 = property class="Str"(reference=w343, "Value"=w342) -> ()  [unwired: 1 in, 2 out]
                }
                n72 = Build Array (concatenate)(w331, w323) -> (w341:dbl[])
                n73 = call "TempPreRunGraph_DP_Ver1.0.vi"("T Array"=w330, "Temp Display Cluster (Need RMS)"=w319, "Set Pt"=w329, "Delta T"=w328) -> ("Temp Graph"=w320:dbl[][])  [unwired: 3 in]
              }
            }
            "T Set Pt (K)" <- w167
            "T Rate (K/min)" <- w166
            "Temp Display Cluster" <- w164
            "Temp Graph" <- w165
            n74 = Tick Count (ms)() -> (millisecond timer value=w187:u32)
            n75 = Equal To 0?(x=w178) -> (x = 0?=w188:bool)
            n76 = Multiply(x=w138, y=u32 60) -> (x*y=w181:u32)
            n77 = case shown="True" w188 {
              tunnel: w187 -> [w345 w348]
              tunnel: [w346 0] -> w189
              frame False {
                n78 = local read "StartTime"() -> (w344:u32)
                n79 = Subtract(x=w345, y=w344) -> (x-y=w346:u32)
              }
              frame True {
                "StartTime" <- w348
              }
            }
            n80 = expression code="x/1000"(w189) -> (w183:u32)
            n81 = Bundle(w153) -> (→"BField Display Cluster":cluster{dbl})  [unwired: 1 in]
            n82 = Quotient & Remainder(x=w183, y=u32 60) -> (x-y*floor(x/y)=w185:u32, floor(x/y)=w186:u32)
            n83 = Greater Or Equal?(x=w183, y=w181) -> (x >= y?=w180:bool)
            n84 = Format Into String(format string="%02d : %02d", w186, w185) -> (resulting string=→"Time 2":string)  [unwired: 2 in, 1 out]
            n85 = And(x=w145, y=w146) -> (x .and. y?=→"Reach to set pt?":bool)
            n86 = Wait (ms)(milliseconds to wait=u32 1000) -> ()  [unwired: 1 out]
            n87 = Compound Arithmetic op=OR("Skip", w180, w146) -> (w144:bool)
            n88 = Or(x=w144, y=w145) -> (x .or. y?=w142:bool)
            n89 = And(x=w144, y=w145) -> (x .and. y?=w143:bool)
            n90 = Select(t=w142, s=w140, f=w143) -> (s? t:f=w141:bool)
          }
          n91 = case shown="False" w94 {
            tunnel: [w122 w128] -> w107
            tunnel: w106 -> [w122 w127]
            tunnel: w105 -> [_ w126]
            tunnel: w104 -> [_ w124]
            tunnel: w103 -> [_ w123]
            frame False {
            }
            frame True {
              n92 = call "IPS120_CloseHeater.vi"("Instrument address (in)"=w124, "Last run?"="Last run?", "B field Change?"=w126, "error in"=w127, "Hold(min)"=w123) -> ("error out"=w128:errorcluster)
            }
          }
        }
      }
      n93 = Cluster To Array(cluster=w43) -> (array=w87:bool[])
      n94 = Build Array("ChB_K" ("f"), "ChC_K" ("f"), "ChD_K" ("f")) -> (w83:string[])
      n95 = for {
        tunnel: w87 -> [w352] mode=indexing
        shift-right: [w349] -> w82
        shift-left: w73 -> [w350]
        tunnel: w83 -> [w351] mode=indexing
        n96 = case shown="False" w352 {
          tunnel: w351 -> [_ w356]
          tunnel: w350 -> [w353 w355]
          tunnel: [w353 w354] -> w349
          frame False {
          }
          frame True {
            n97 = Build Array (concatenate)(w355, w356) -> (w354:string[])
          }
        }
      }
      n98 = Build Array("T1_K" ("element"), "T2_K" ("f"), "T3_K" ("f")) -> (w75:string[])
      n99 = Build Array (concatenate)(w81, w82) -> (w80:string[])
      n100 = Build Array("BField_T" ("f")) -> (w71:string[])
      n101 = Select(t=w73, s=w63, f=w80) -> (s? t:f=w79:string[])
      n102 = Select(t=w73, s=w58, f=w75) -> (s? t:f=w74:string[])
      n103 = Select(t=w73, s=w50, f=w71) -> (s? t:f=w70:string[])
      n104 = Build Array (concatenate)(w79, w74, w70) -> (w78:string[])
      n105 = Concatenate Strings("No magnetic field in this measurment.", "\r\n") -> (w49:string)
      n106 = Concatenate Strings("With magnet. The field will be recorded in unit of Tesla.", "\r\n") -> (w48:string)
      n107 = Select(t=w49, s=w50, f=w48) -> (s? t:f=w45:string)
      n108 = Concatenate Strings("ITC 503 attched. T1, T2 and T3 will be recorded. Corresponding to the T1, T2 and T3 columns. T will be recorded in unit of K. ", "\r\n") -> (w56:string)
      n109 = Concatenate Strings("Lakeshore 340 attched. T will be recorded in unit of K. ", "\r\n") -> (w61:string)
      n110 = Select(t="", s=w58, f=w56) -> (s? t:f=w46:string)
      n111 = Select(t="", s=w63, f=w61) -> (s? t:f=w47:string)
      n112 = Concatenate Strings(w47, w46, w45) -> (w44:string)
    }
    frame True {
      # "Temp. and B-field are both not controled"
      n113 = Concatenate Strings("Neither Temp nor B-field is not controlled", "\r\n") -> (w357:string)
    }
  }
  "Comments String" <- w19
  n114 = Build Array (concatenate)("Time_sec", w29) -> (→"Title Array":string[])
  n115 = Merge Errors(w25, w24) -> (→"error out":errorcluster)
  "output cluster 2" <- "output cluster"
